vi "Read Voltage.vi"(6 "Error In":errorcluster) -> (0 "Error Out":errorcluster, 3 "Voltage":dbl)   [LabVIEW 2025]
doc: "This VI is used in the LabVIEW Core 1 & 2 courses.\n\nThis VI simulates taking voltage readings from a DAQ board. Use this VI to replace the DAQ Assistant Express VI in any temperature reading exercises in this course. This VI is used as a subVI in all (Demo) exercises."
panel:
  # "This VI is a demo version of a VI that reads the voltage on Device 1, channel 0.  When scaled by 100, value can represent temperature."
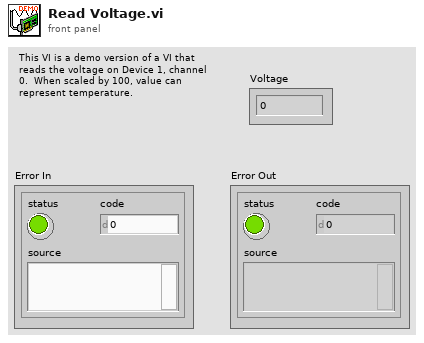
[diagram p1: front panel]
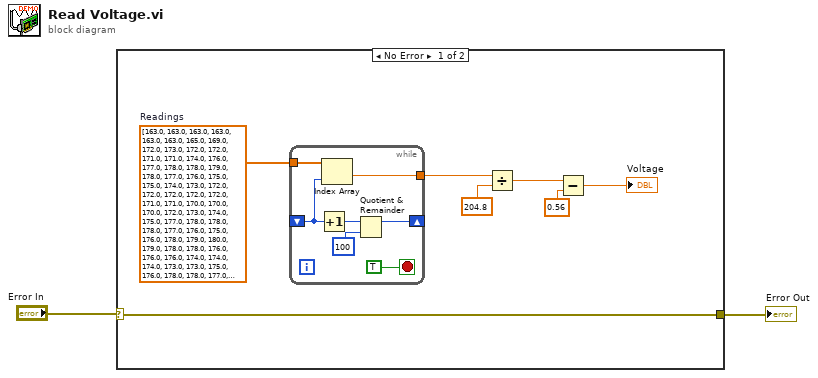
[diagram p0: block diagram]
diagram:
  n1 = case shown="No Error" "Error In" {
    selector: "Error In" -> [w5 w17]
    tunnel: [w5 w17] -> w2
    frame No Error {
      w3 = dbl[] [163.0, 163.0, 163.0, 163.0, 163.0, 163.0, 165.0, 169.0, 172.0, 173.0, 172.0, 172.0, 171.0, 171.0, 174.0, 176.0, 177.0, 178.0, 178.0, 179.0, 178.0, 177.0, 176.0, 175.0, 175.0, 174.0, 173.0, 172.0, 172.0, 172.0, 172.0, 172.0, 171.0, 171.0, 170.0, 170.0, 170.0, 172.0, 173.0, 174.0, 175.0, 177.0, 178.0, 178.0, 178.0, 177.0, 176.0, 175.0, 176.0, 178.0, 179.0, 180.0, 179.0, 178.0, 178.0, 176.0, 176.0, 176.0, 174.0, 174.0, 174.0, 173.0, 173.0, 175.0, 176.0, 178.0, 178.0, 177.0, 176.0, 175.0, 175.0, 174.0, 174.0, 173.0, 173.0, 172.0, 172.0, 171.0, 171.0, 170.0, 170.0, 170.0, 170.0, 170.0, 170.0, 170.0, 169.0, 166.0, 167.0, 169.0, 170.0, 169.0, 168.0, 168.0, 168.0, 168.0, 167.0, 167.0, 167.0, 167.0]  # Readings
      n2 = while {
        tunnel: w3 -> [w11]
        tunnel: [w12] -> w8
        shift-left: _ -> [w16]
        shift-right: [w13] -> _
        stop <- TRUE stop-if-true
        n3 = Increment(x=w16) -> (x+1=w15:i32)
        n4 = Index Array(array=w11, index=w16) -> (element=w12:dbl)
        n5 = Quotient & Remainder(x=w15, y=100) -> (x-y*floor(x/y)=w13:i32)  [unwired: 1 out]
      }
      n6 = Divide(x=w8, y=204.8) -> (x/y=w7:dbl)
      n7 = Subtract(x=w7, y=0.56) -> (x-y=→"Voltage":dbl)
    }
    frame Error {
    }
  }
  "Error Out" <- w2
